vi "empty queue.vi"(8 "error in (no error)":errorcluster, 11 "Queue in":refnum<queue>) -> (3 "Queue emptied?":bool)   [LabVIEW 2014]
uses:
  experimental data.ctl
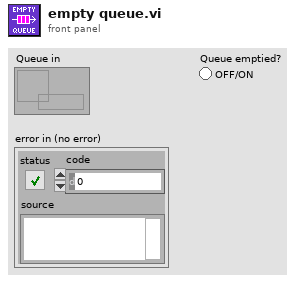
[diagram p1: front panel]
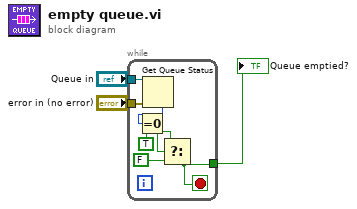
[diagram p0: block diagram]
diagram:
  n1 = while {
    tunnel: "error in (no error)" -> [w10]
    tunnel: "Queue in" -> [w9]
    tunnel: [w4] -> w3
    stop <- w4 stop-if-true
    n2 = Get Queue Status(queue=w9, error in (no error)=w10) -> (# elements in queue=w8:i32)  [unwired: 1 in, 7 out]
    n3 = Equal To 0?(x=w8) -> (x = 0?=w7:bool)
    n4 = Select(t=TRUE, s=w7, f=FALSE) -> (s? t:f=w4:bool)
  }
  "Queue emptied?" <- w3
